vi "3-5 case structure.vi"() -> ()   [LabVIEW 2015]
doc: "This simple VI thorws a warning if the Current temp input is greater than the max temp input or less than the min temp input."
panel:
  out "Warning?":bool
  out "Warning Text":string
  in  "Max Temp":dbl=30.0
  in  "Min Temp":dbl=10.0
  in  "Current Temp":dbl=25.0
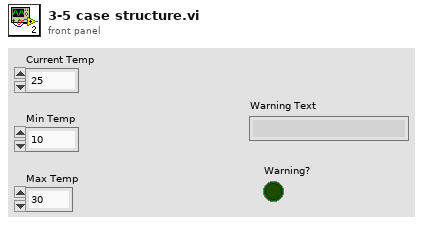
[diagram p1: front panel]
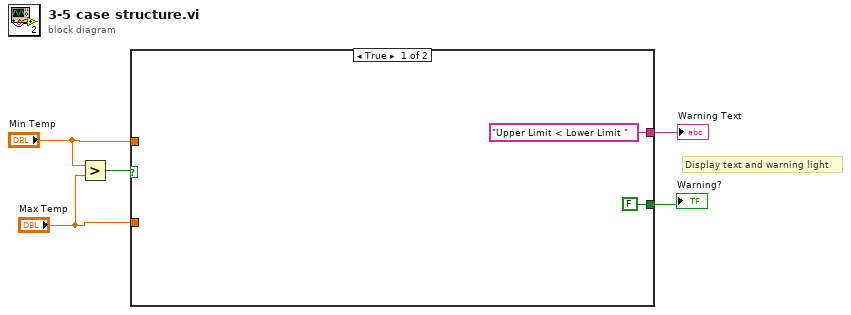
[diagram p0: block diagram]
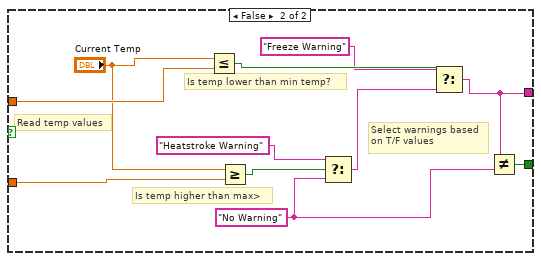
[diagram p2: hidden frame]
diagram:
  # "Display text and warning light"
  n1 = Greater?(x="Min Temp", y="Max Temp") -> (0:w1:bool)
  n2 = case shown="True" w1 {
    tunnel: "Max Temp" -> [_ w18]
    tunnel: "Min Temp" -> [_ w17]
    tunnel: ["Upper Limit < Lower Limit " w9] -> w5
    tunnel: [FALSE w8] -> w4
    frame True {
    }
    frame False {
      w10 = "No Warning"
      # "Read temp values"
      # "Select warnings based\non T/F values"
      # "Is temp higher than max>"
      # "Is temp lower than min temp?"
      n3 = Less Or Equal?(x="Current Temp", y=w17) -> (x <= y?=w15:bool)
      n4 = Greater Or Equal?(x="Current Temp", y=w18) -> (x >= y?=w14:bool)
      n5 = Select(t="Heatstroke Warning", s=w14, f=w10) -> (s? t:f=w11:string)
      n6 = Select(t="Freeze Warning", s=w15, f=w11) -> (s? t:f=w9:string)
      n7 = Not Equal?(x=w9, y=w10) -> (x != y?=w8:bool)
    }
  }
  "Warning Text" <- w5
  "Warning?" <- w4
